vi "X-_Tx_Rx_strip_echo.vi"(4 "Terminate Count":i32, 5 "Channel Name":string, 6 "Write String":string, 7 "Iteration No":i32, 8 "Port Name":string) -> (0 "Non-Blank reply":bool, 1 "Good Echo":bool, 3 "Reply":string)   [LabVIEW 2010]
panel:
  out "Read String":string
  out "Echo Found":string
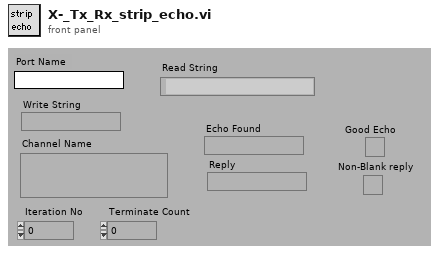
[diagram p1: front panel]
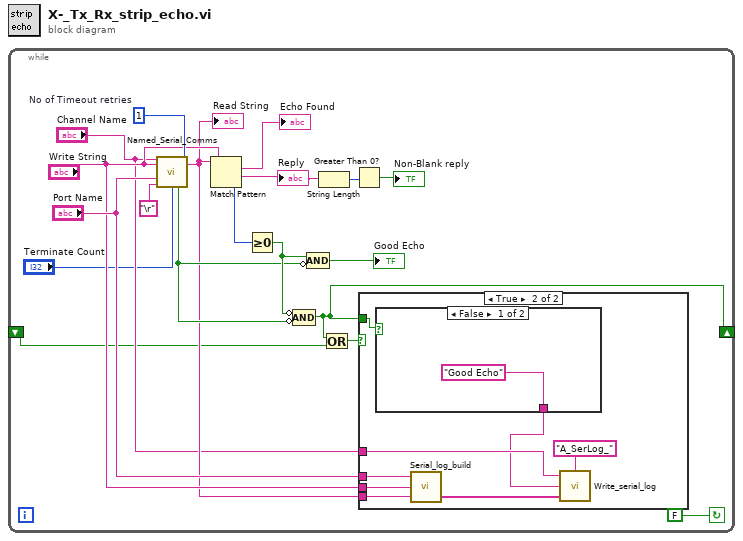
[diagram p0: block diagram]
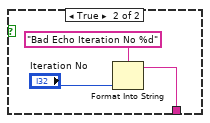
[diagram p3: hidden frame]
diagram:
  n1 = while {
    shift-left: _ -> [w6]
    shift-right: [w4] -> _
    stop <- FALSE continue-if-true
    w17 = 1  # No of Timeout retries
    n2 = call "Named_Serial_Comms.vi"("Channel Name"="Channel Name", "Write String"="Write String", "!Timeout retries"=w17, "Port Name"="Port Name", "Term Grep"="\r", "Terminate Count"="Terminate Count") -> ("Read"=w8:string, "Timed out"=w11:bool)  [unwired: 3 in, 5 out]
    "Read String" <- w8
    n3 = Match Pattern(string=w8, regular expression="Write String") -> (match substring=→"Echo Found":string, after substring=w15:string, offset past match=w19:i32)  [unwired: 2 out]
    "Reply" <- w15
    n4 = Greater Or Equal To 0?(x=w19) -> (x >= 0?=w12:bool)
    n5 = Compound Arithmetic op=AND(invert w12, invert w11) -> (w4:bool)
    n6 = Compound Arithmetic op=AND(w12, invert w11) -> (→"Good Echo":bool)
    n7 = String Length(string=w15) -> (length=w16:i32)
    n8 = Or(x=w4, y=w6) -> (x .or. y?=w5:bool)
    n9 = Greater Than 0?(x=w16) -> (x > 0?=→"Non-Blank reply":bool)
    n10 = case shown="True" w5 {
      tunnel: "Port Name" -> [_ w26]
      tunnel: "Write String" -> [_ w27]
      tunnel: w8 -> [_ w25]
      tunnel: "Channel Name" -> [_ w23]
      tunnel: w4 -> [_ w21]
      frame False {
      }
      frame True {
        n11 = case shown="False" w21 {
          tunnel: ["Good Echo" ("Header message") w29] -> w20
          frame False {
          }
          frame True {
            n12 = Format Into String(format string="Bad Echo Iteration No %d" ("Format String"), "Iteration No") -> (resulting string=w29:string)  [unwired: 2 in, 1 out]
          }
        }
        n13 = call "Serial_log_build.vi"("Read"=w25, "Write String"=w27, "Port Name"=w26) -> ("Output Array"=w22:string[])
        n14 = call "Write_serial_log.vi"("Log Type"="A_SerLog_", "Log Array"=w22, "Header message"=w20, "Channel Name"=w23) -> ()  [unwired: 1 out]
      }
    }
  }
